vi "Generate Waveform.vi"(0 "signal configuration":refnum<class "SV Noise.lvclass">, 5 "template waveform":waveform(dbl), 9 "samples":i32, 11 "error in (no error)":errorcluster) -> (4 "signal configuration":refnum<class "SV Noise.lvclass">, 6 "output waveform":waveform(dbl), 10 "samples":i32, 15 "error out":errorcluster)   [LabVIEW 2017, in "SV Noise.lvclass"]
uses:
  <vilib>/addons/_NISVFA/_Generation/Signal Generation/SV Noise/SV Noise.lvclass
  C:/Program Files (x86)/National Instruments/LabVIEW 2017/vi.lib/addons/_NISVFA/_Generation/Signal Generation/SV Signal/SV Signal.lvclass
  <vilib>/addons/_NISVFA/_Generation/Signal Generation/SV Signal/SV Signal.lvclass/SV Signal.ctl
  <vilib>/addons/_NISVFA/_Generation/Signal Generation/SV Noise/SV Noise.lvclass/SV Noise.ctl
  <vilib>/addons/_NISVFA/_Generation/Signal Generation/SV Signal/Read Sample Rate.vi
  <vilib>/Analysis/NI_AALBase.lvlib
  <vilib>/addons/_NISVFA/_Generation/Signal Generation/SV Signal/SV Signal.lvclass
  <vilib>/addons/_NISVFA/_Generation/SoundVib_Generation.lvlib
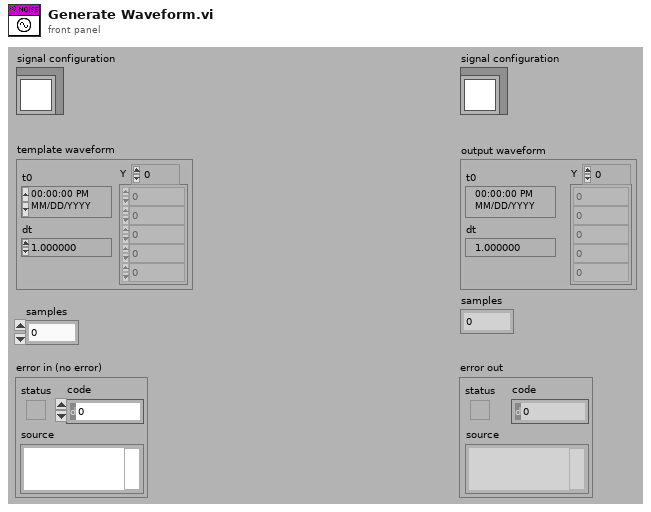
[diagram p1: front panel]
types:
  T1 = enum16{"White noise", "Pink noise", "Periodic random noise"}
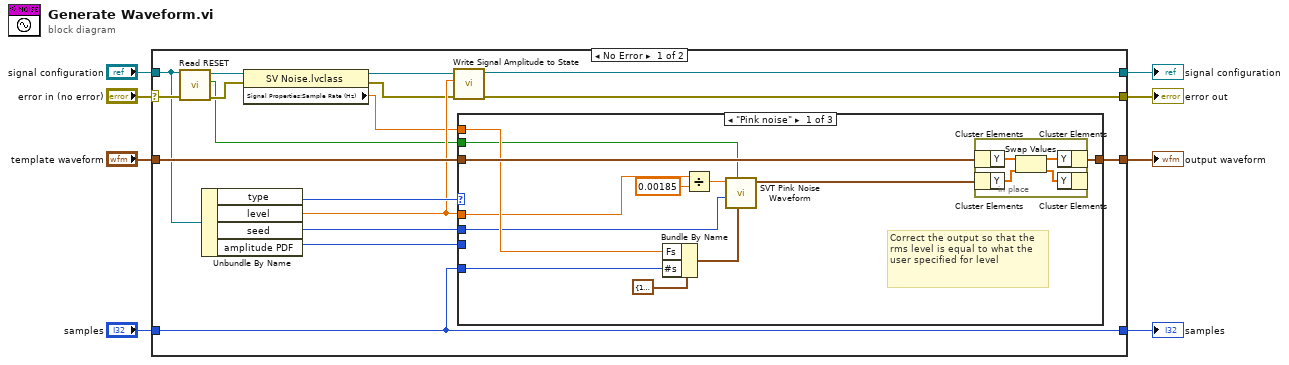
[diagram p0: block diagram]
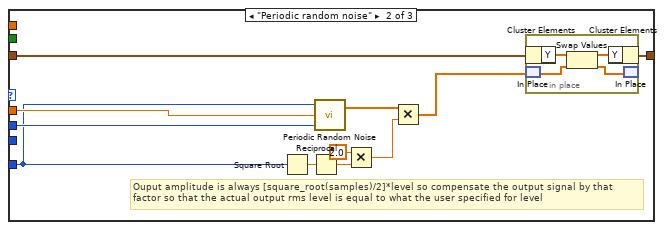
[diagram p2: hidden frame]
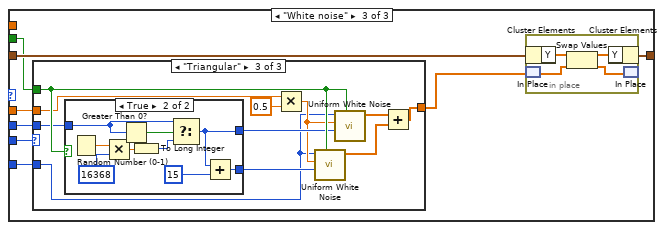
[diagram p3: hidden frame]
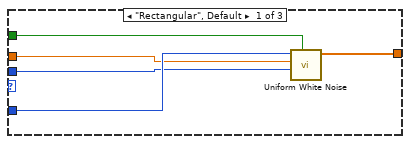
[diagram p4: hidden frame]
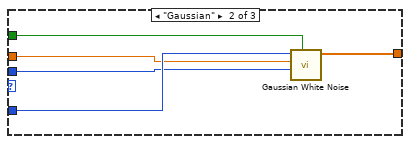
[diagram p5: hidden frame]
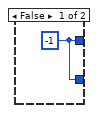
[diagram p6: hidden frame]
diagram:
  n1 = case shown="No Error" "error in (no error)" {
    selector: "error in (no error)" -> [w13 w102]
    tunnel: [w17 w102] -> w7
    tunnel: [w19 w101] -> w5
    tunnel: "signal configuration" -> [w11 w101]
    tunnel: [w24 w100] -> w4
    tunnel: [w23 _] -> w3
    tunnel: "samples" -> [w23 _]
    tunnel: "template waveform" -> [w22 w100]
    frame No Error {
      n2 = call <vilib>:"Read RESET.vi"("error in (no error)"=w13, "SV Signal in"=w11) -> ("error out"=w12:errorcluster, "RESET"=w9:bool, "SV Signal out"=w10:refnum<class "SV Noise.lvclass">)  [unwired: 7 in]
      n3 = Unbundle By Name(w11) -> ("type"=w25:T1, "level"=w18:dbl, "seed"=w21:i32, "amplitude PDF"=w20:enum16{"Gaussian", "Rectangular", "Triangular"})
      n4 = property class="SV Noise.lvclass"(reference=w10, error in=w12) -> (reference out=w16:refnum<class "SV Noise.lvclass">, error out=w15:errorcluster, "Signal Properties:Sample Rate (Hz)"=w14:dbl)
      n5 = call <vilib>:"Write Signal Amplitude to State.vi"("error in (no error)"=w15, "amplitude"=w18, "SV Signal in"=w16) -> ("error out"=w17:errorcluster, "SV Signal out"=w19:refnum<class "SV Noise.lvclass">)  [unwired: 7 in]
      n6 = case shown="\"Pink noise\"" w25 {
        tunnel: w22 -> [w35 w52 w64]
        tunnel: w18 -> [w27 w51 w62]
        tunnel: w23 -> [w34 w48 w61]
        tunnel: [w37 w50 w60] -> w24
        tunnel: w21 -> [w28 w49 w59]
        tunnel: w9 -> [w30 _ w58]
        tunnel: w20 -> [_ _ w57]
        tunnel: w14 -> [w33 _ _]
        frame "Pink noise" {
          # "Correct the output so that the rms level is equal to what the user specified for level"
          n7 = Bundle By Name(cluster=cluster{"Fs":dbl, "#s":dbl} {"Fs"=1000.0, "#s"=1000.0} ("sampling info"), "Fs"=w33, "#s"=w34) -> (w29:cluster{"Fs":dbl, "#s":dbl})
          n8 = Divide(x=w27, y=0.00185 ("ratio of level to amplitude")) -> (x/y=w31:dbl)
          n9 = call <vilib>:"SVT Pink Noise Waveform.vi"("sampling info"=w29, "reset signal (F)"=w30, "seed"=w28, "amplitude"=w31) -> ("pink noise signal"=w26:waveform(dbl))  [unwired: 6 in, 1 out]
          n10 = in-place {
            n11 = in-place-cluster #1(w35) -> ("Y"=w41:dbl[])
            n12 = in-place-cluster #2(w26) -> ("Y"=w39:dbl[])
            n13 = Swap Values(12:w41, 14:w39) -> (1:w40:dbl[], 3:w38:dbl[])  [unwired: 1 in]
            n14 = in-place-cluster #1("Y"=w40) -> (w37:waveform(dbl))
            n15 = in-place-cluster #2("Y"=w38) -> ()  [unwired: 1 out]
          }
        }
        frame "Periodic random noise" {
          # "Ouput amplitude is always [square_root(samples)/2]*level so compensate the output signal by that factor so that the actual output rms level is equal to what the user specified for level"
          n16 = Square Root(x=w48) -> (sqrt(x)=w47:dbl)
          n17 = Reciprocal(x=w47) -> (1/x=w46:dbl)
          n18 = call <vilib>:"Periodic Random Noise.vi"("seed"=w49, "spectral amplitude"=w51, "samples"=w48) -> ("periodic random noise"=w44:dbl[])  [unwired: 1 out]
          n19 = Multiply(x=2.0, y=w46) -> (x*y=w43:dbl)
          n20 = Multiply(x=w44, y=w43) -> (x*y=w42:dbl[])
          n21 = in-place {
            n22 = in-place-cluster #3(w52) -> ("Y"=w56:dbl[])
            n23 = in-place-match #4(w42) -> (w54:dbl[])
            n24 = Swap Values(12:w56, 14:w54) -> (1:w55:dbl[], 3:w53:dbl[])  [unwired: 1 in]
            n25 = in-place-cluster #3("Y"=w55) -> (w50:waveform(dbl))
            n26 = in-place-match #4(w53) -> ()  [unwired: 1 out]
          }
        }
        frame "White noise" {
          n27 = case shown="\"Triangular\"" w57 {
            tunnel: w61 -> [w69 w74 w75]
            tunnel: [w68 w73 w80] -> w63
            tunnel: w62 -> [w67 w72 w78]
            tunnel: w58 -> [w66 w71 w83]
            tunnel: w59 -> [w65 w70 w81]
            frame "Rectangular", Default {
              n28 = call <vilib>:"Uniform White Noise.vi"("initialize?"=w66, "seed"=w65, "amplitude"=w67, "samples"=w69) -> ("uniform white noise"=w68:dbl[])  [unwired: 6 in, 1 out]
            }
            frame "Gaussian" {
              n29 = call <vilib>:"Gaussian White Noise.vi"("initialize?"=w71, "seed"=w70, "standard deviation"=w72, "samples"=w74) -> ("Gaussian noise pattern"=w73:dbl[])  [unwired: 6 in, 1 out]
            }
            frame "Triangular" {
              n30 = case shown="True" w83 {
                tunnel: [w86 w89] -> w82
                tunnel: w81 -> [_ w88]
                tunnel: [w86 w87] -> w79
                frame False {
                  w86 = -1 ("seed")
                }
                frame True {
                  n31 = Random Number (0-1)() -> (number: 0 to 1=w93:dbl)
                  n32 = Multiply(x=w93, y=16368 ("x")) -> (x*y=w94:dbl)
                  n33 = Greater Than 0?(x=w88) -> (x > 0?=w95:bool)
                  n34 = To Long Integer(number=w94) -> (32bit integer=w91:i32)
                  n35 = Select(t=w88, s=w95, f=w91) -> (s? t:f=w87:i32)
                  n36 = Add(x=w87, y=15) -> (x+y=w89:i32)
                }
              }
              n37 = Multiply(x=w78, y=0.5) -> (x*y=w76:dbl)
              n38 = call <vilib>:"Uniform White Noise.vi"("initialize?"=w83, "seed"=w82, "amplitude"=w76, "samples"=w75) -> ("uniform white noise"=w85:dbl[])  [unwired: 6 in, 1 out]
              n39 = call <vilib>:"Uniform White Noise.vi"("initialize?"=w83, "seed"=w79, "amplitude"=w76, "samples"=w75) -> ("uniform white noise"=w84:dbl[])  [unwired: 6 in, 1 out]
              n40 = Add(x=w84, y=w85) -> (x+y=w80:dbl[])
            }
          }
          n41 = in-place {
            n42 = in-place-cluster #5(w64) -> ("Y"=w99:dbl[])
            n43 = in-place-match #6(w63) -> (w97:dbl[])
            n44 = Swap Values(12:w99, 14:w97) -> (1:w98:dbl[], 3:w96:dbl[])  [unwired: 1 in]
            n45 = in-place-cluster #5("Y"=w98) -> (w60:waveform(dbl))
            n46 = in-place-match #6(w96) -> ()  [unwired: 1 out]
          }
        }
      }
    }
    frame Error {
    }
  }
  "error out" <- w7
  "signal configuration" <- w5
  "output waveform" <- w4
  "samples" <- w3
